vi "Init Log.vi"(8 "error in (no error)":errorcluster, 11 "GuiderSetup in":refnum<class "GuiderSetup.lvclass">) -> (0 "error out":errorcluster, 3 "GuiderSetup out":refnum<class "GuiderSetup.lvclass">)   [LabVIEW 2018, in "GuiderSetup.lvclass"]
uses:
  GuiderSetup.lvclass
  C:/Users/devstaff/sparc4/s4gui/Versao ZeroMQ REQ-REP/SPARC4_GUI -v1.0.0 - 20250116/S4GUI/S4GUI.lvclass
  S4GUI/S4GUI.lvclass/S4GUI.ctl
  GuiderSetup.lvclass/GuiderSetup.ctl
  Instrument/Instrument.lvclass
  Log/Log.lvclass
  PublisherGS/PublisherGS.lvclass
  AG/AG.lvclass
  Comm/Stream/Stream.lvclass
  S4GUI/S4GUI.lvclass
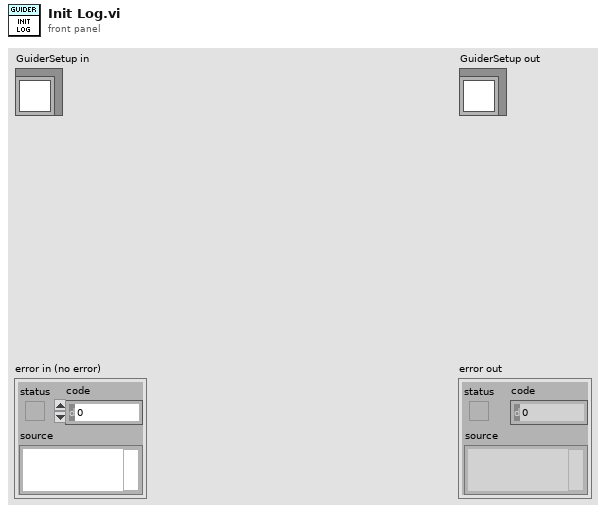
[diagram p1: front panel]
types:
  T1 = enum16{"open", "replace", "create", "open or create", "replace or create", "replace or create with confirmation"}
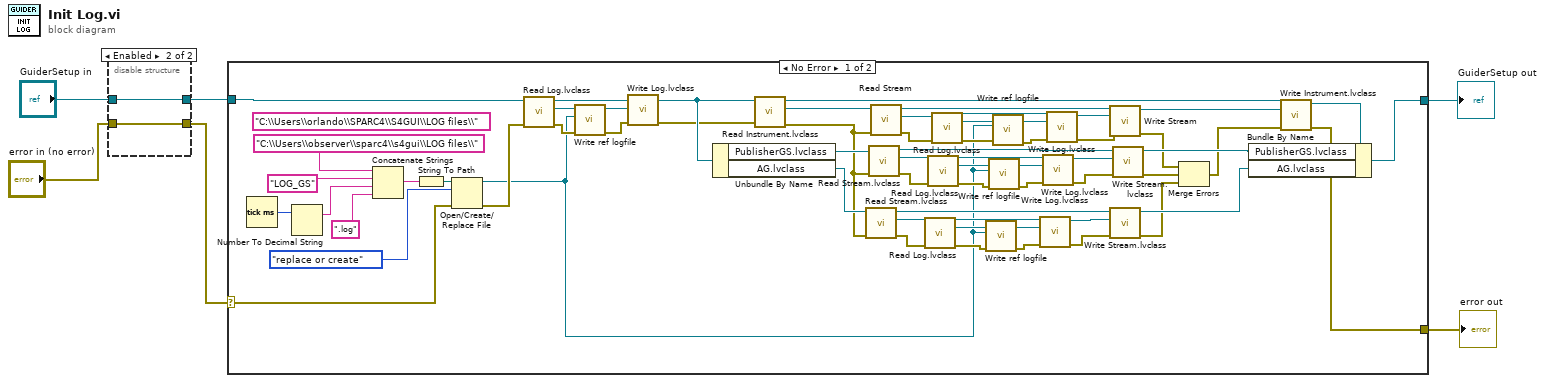
[diagram p0: block diagram]
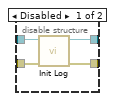
[diagram p2: hidden frame]
diagram:
  n1 = disable-structure shown="Enabled" {
    disable-tunnel: "error in (no error)" -> [w10 w11]
    disable-tunnel: "GuiderSetup in" -> [w9 w12]
    disable-tunnel: [w8 w12] -> w4
    disable-tunnel: [w7 w11] -> w2
    frame Disabled {
      n2 = call-parent "Init Log.vi"("error in (no error)"=w10, "S4GUI in"=w9) -> ("error out"=w7:errorcluster, "S4GUI out"=w8:refnum<class "GuiderSetup.lvclass">)  [unwired: 8 in]
    }
    frame Enabled {
    }
  }
  n3 = case shown="No Error" w2 {
    selector: w2 -> [w62 w77]
    tunnel: w4 -> [w69 w78]
    tunnel: [w50 w78] -> w3
    tunnel: [w15 w77] -> w1
    frame No Error {
      (unwired) "C:\\Users\\orlando\\SPARC4\\S4GUI\\LOG files\\"
      n4 = Tick Count (ms)() -> (millisecond timer value=w71:u32)
      n5 = Number To Decimal String(number=w71) -> (decimal integer string=w70:string)  [unwired: 1 in]
      n6 = Concatenate Strings("C:\\Users\\observer\\sparc4\\s4gui\\LOG files\\" ("string"), "LOG_GS" ("string"), w70, ".log" ("string")) -> (w74:string)
      n7 = String To Path(string=w74) -> (path=w75:path)
      n8 = Open/Create/Replace File(file path (use dialog)=w75, error in=w62, operation (0:open)=T1."replace or create") -> (refnum out=w14:refnum<file>, error out=w65:errorcluster)  [unwired: 3 in, 1 out]
      n9 = call-dynamic "Read Log.lvclass.vi"("error in (no error)"=w65, "S4GUI in"=w69) -> ("error out"=w64:errorcluster, "Log.lvclass"=w68:refnum<class "Log.lvclass">, "S4GUI out"=w67:refnum<class "GuiderSetup.lvclass">)  [unwired: 7 in]
      n10 = call-dynamic "Write ref logfile.vi"("error in (no error)"=w64, "ref logfile"=w14, "Log in"=w68) -> ("error out"=w63:errorcluster, "Log out"=w66:refnum<class "Log.lvclass">)  [unwired: 7 in]
      n11 = call-dynamic "Write Log.lvclass.vi"("error in (no error)"=w63, "Log.lvclass"=w66, "S4GUI in"=w67) -> ("error out"=w18:errorcluster, "S4GUI out"=w34:refnum<class "GuiderSetup.lvclass">)  [unwired: 7 in]
      n12 = Unbundle By Name(w34) -> ("PublisherGS.lvclass"=w58:refnum<class "PublisherGS.lvclass">, "AG.lvclass"=w39:refnum<class "AG.lvclass">)
      n13 = call "Read Instrument.lvclass.vi"("error in (no error)"=w18, "S4ACS_GUI in"=w34) -> ("error out"=w17:errorcluster, "Instrument.lvclass"=w31:refnum<class "Instrument.lvclass">, "S4ACS_GUI out"=w33:refnum<class "GuiderSetup.lvclass">)  [unwired: 7 in]
      n14 = call-dynamic "Read Stream.lvclass.vi"("error in (no error)"=w17, "Client in"=w39) -> ("error out"=w43:errorcluster, "Stream.lvclass"=w46:refnum<class "Stream.lvclass">, "Client out"=w44:refnum<class "AG.lvclass">)  [unwired: 7 in]
      n15 = call-dynamic "Read Stream.lvclass.vi"("error in (no error)"=w17, "Client in"=w58) -> ("error out"=w54:errorcluster, "Stream.lvclass"=w57:refnum<class "Stream.lvclass">, "Client out"=w55:refnum<class "PublisherGS.lvclass">)  [unwired: 7 in]
      n16 = call-dynamic "Read Stream.vi"("error in (no error)"=w17, "Server in"=w31) -> ("error out"=w23:errorcluster, "Stream.lvclass"=w25:refnum<class "Stream.lvclass">, "Server out"=w30:refnum<class "Instrument.lvclass">)  [unwired: 7 in]
      n17 = call-dynamic "Read Log.lvclass.vi"("error in (no error)"=w43, "Comm in"=w46) -> ("error out"=w42:errorcluster, "Log.lvclass"=w49:refnum<class "Log.lvclass">, "Comm out"=w48:refnum<class "Stream.lvclass">)  [unwired: 7 in]
      n18 = call-dynamic "Read Log.lvclass.vi"("error in (no error)"=w54, "Comm in"=w57) -> ("error out"=w53:errorcluster, "Log.lvclass"=w61:refnum<class "Log.lvclass">, "Comm out"=w60:refnum<class "Stream.lvclass">)  [unwired: 7 in]
      n19 = call-dynamic "Read Log.lvclass.vi"("error in (no error)"=w23, "Comm in"=w25) -> ("error out"=w22:errorcluster, "Log.lvclass"=w28:refnum<class "Log.lvclass">, "Comm out"=w27:refnum<class "Stream.lvclass">)  [unwired: 7 in]
      n20 = call-dynamic "Write ref logfile.vi"("error in (no error)"=w42, "ref logfile"=w14, "Log in"=w49) -> ("error out"=w41:errorcluster, "Log out"=w47:refnum<class "Log.lvclass">)  [unwired: 7 in]
      n21 = call-dynamic "Write ref logfile.vi"("error in (no error)"=w53, "ref logfile"=w14, "Log in"=w61) -> ("error out"=w52:errorcluster, "Log out"=w59:refnum<class "Log.lvclass">)  [unwired: 7 in]
      n22 = call-dynamic "Write ref logfile.vi"("error in (no error)"=w22, "ref logfile"=w14, "Log in"=w28) -> ("error out"=w21:errorcluster, "Log out"=w26:refnum<class "Log.lvclass">)  [unwired: 7 in]
      n23 = call-dynamic "Write Log.lvclass.vi"("error in (no error)"=w41, "Log.lvclass"=w47, "Comm in"=w48) -> ("error out"=w40:errorcluster, "Comm out"=w45:refnum<class "Stream.lvclass">)  [unwired: 7 in]
      n24 = call-dynamic "Write Log.lvclass.vi"("error in (no error)"=w52, "Log.lvclass"=w59, "Comm in"=w60) -> ("error out"=w51:errorcluster, "Comm out"=w56:refnum<class "Stream.lvclass">)  [unwired: 7 in]
      n25 = call-dynamic "Write Log.lvclass.vi"("error in (no error)"=w21, "Log.lvclass"=w26, "Comm in"=w27) -> ("error out"=w20:errorcluster, "Comm out"=w24:refnum<class "Stream.lvclass">)  [unwired: 7 in]
      n26 = call-dynamic "Write Stream.vi"("error in (no error)"=w20, "Stream.lvclass"=w24, "Server in"=w30) -> ("error out"=w19:errorcluster, "Server out"=w29:refnum<class "Instrument.lvclass">)  [unwired: 7 in]
      n27 = call-dynamic "Write Stream.lvclass.vi"("error in (no error)"=w40, "Stream.lvclass"=w45, "Client in"=w44) -> ("error out"=w35:errorcluster, "Client out"=w38:refnum<class "AG.lvclass">)  [unwired: 7 in]
      n28 = call-dynamic "Write Stream.lvclass.vi"("error in (no error)"=w51, "Stream.lvclass"=w56, "Client in"=w55) -> ("error out"=w36:errorcluster, "Client out"=w37:refnum<class "PublisherGS.lvclass">)  [unwired: 7 in]
      n29 = Merge Errors(w19, w36, w35) -> (w16:errorcluster)
      n30 = call "Write Instrument.lvclass.vi"("error in (no error)"=w16, "Instrument.lvclass"=w29, "S4ACS_GUI in"=w33) -> ("error out"=w15:errorcluster, "S4ACS_GUI out"=w32:refnum<class "GuiderSetup.lvclass">)  [unwired: 7 in]
      n31 = Bundle By Name(cluster=w32, "PublisherGS.lvclass"=w37, "AG.lvclass"=w38) -> (w50:refnum<class "GuiderSetup.lvclass">)
    }
    frame Error {
    }
  }
  "error out" <- w1
  "GuiderSetup out" <- w3
